vi "Transform Assemby into Channel List.vi"(11 "Assembly Configuration":T3[](array[typedef])) -> (3 "Channel Configuration":T1[](array[typedef]))   [LabVIEW 2023, in "Ethernet IP Custom Device Custom Device.lvlib"]
uses:
  Ethernet IP Custom Device Custom Device.lvlib
  EIP Attribute Tag Configuration.ctl
  EIP Attribute Direction.ctl
  EIP Attribute Channel Info.ctl
  assembly map key.ctl
  assembly map value.ctl
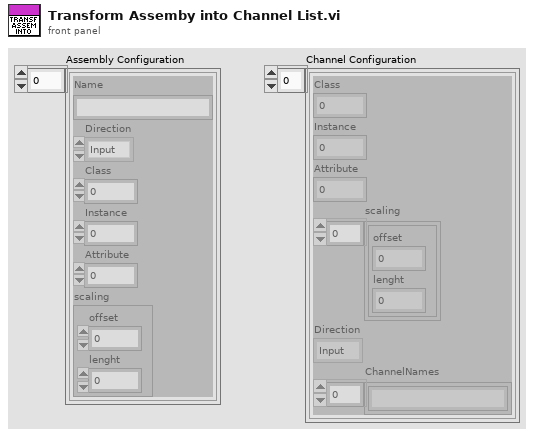
[diagram p1: front panel]
types:
  T1 = typedef "Ethernet IP Custom Device Custom Device.lvlib/EIP Attribute Channel Info.ctl" = cluster{"Class":i32, "Instance":u32, "Attribute":i32, "scaling":cluster{"offset":u32, "lenght":u32}[], "Direction":T2, "ChannelNames":string[]}
  T2 = typedef "Ethernet IP Custom Device Custom Device.lvlib/EIP Attribute Direction.ctl" = enum16{"Input", "Output"}
  T3 = typedef "Ethernet IP Custom Device Custom Device.lvlib/EIP Attribute Tag Configuration.ctl" = cluster{"Name":string, "Direction":T2, "Class":i32, "Instance":u32, "Attribute":i32, "scaling":cluster{"offset":u32, "lenght":u32}}
  T4 = typedef "Ethernet IP Custom Device Custom Device.lvlib/assembly map key.ctl" = cluster{"Class":i32, "Attribute":i32, "Instance":u32}
  T5 = typedef "Ethernet IP Custom Device Custom Device.lvlib/assembly map value.ctl" = cluster{"Names":string[], "scaling":cluster{"offset":u32, "lenght":u32}[], "direction":T2}
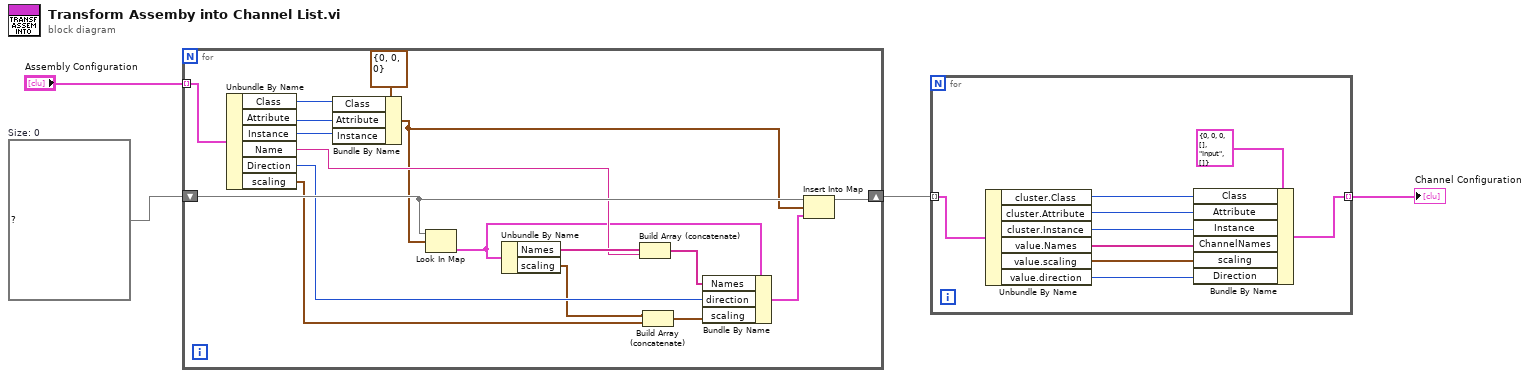
[diagram p0: block diagram]
diagram:
  w3 = map{T4, T5} {}  # Size: 0
  n1 = for {
    tunnel: "Assembly Configuration" -> [w21] mode=indexing
    shift-right: [w16] -> w2
    shift-left: w3 -> [w15]
    n2 = Unbundle By Name(w21) -> ("Class"=w19:i32, "Attribute"=w18:i32, "Instance"=w17:u32, "Name"=w13:string, "Direction"=w10:T2, "scaling"=w8:cluster{"offset":u32, "lenght":u32})
    n3 = Bundle By Name(cluster=T4 {"Class"=0, "Attribute"=0, "Instance"=0}, "Class"=w19, "Attribute"=w18, "Instance"=w17) -> (w5:T4)
    n4 = Look In Map(map=w15, key=w5) -> (value=w12:T5)  [unwired: 1 in, 1 out]
    n5 = Unbundle By Name(w12) -> ("Names"=w14:string[], "scaling"=w9:cluster{"offset":u32, "lenght":u32}[])
    n6 = Build Array (concatenate)(w14, w13) -> (w11:string[])
    n7 = Build Array (concatenate)(w9, w8) -> (w7:cluster{"offset":u32, "lenght":u32}[])
    n8 = Bundle By Name(cluster=w12, "Names"=w11, "direction"=w10, "scaling"=w7) -> (w6:T5)
    n9 = Insert Into Map(map in=w15, key=w5, value=w6) -> (map out=w16:map{T4, T5})  [unwired: 2 out]
  }
  n10 = for {
    tunnel: w2 -> [w28] mode=indexing
    tunnel: [w29] -> w1 mode=indexing
    n11 = Unbundle By Name(w28) -> ("cluster.Class"=w27:i32, "cluster.Attribute"=w23:i32, "cluster.Instance"=w22:u32, "value.Names"=w26:string[], "value.scaling"=w25:cluster{"offset":u32, "lenght":u32}[], "value.direction"=w24:T2)
    n12 = Bundle By Name(cluster=T1 {"Class"=0, "Instance"=0, "Attribute"=0, "scaling"=[], "Direction"=enum."Input", "ChannelNames"=[]} ("Channel Configuration"), "Class"=w27, "Attribute"=w23, "Instance"=w22, "ChannelNames"=w26, "scaling"=w25, "Direction"=w24) -> (w29:T1)
  }
  "Channel Configuration" <- w1
